vi "Camera_QR Code Detection.vi"(8 "error in (no error)":errorcluster, 10 "QR Code Detection":T1, 11 "SRV In":refnum<k5>) -> (0 "error out":errorcluster, 3 "SRV Out":refnum<k5>)   [LabVIEW 2014]
doc: "Enables/disables the QR Code detection.\n\n\nAuthor: Mike Schultz"
uses:
  ImageProcessing/QR Code Detection Radio Buttons.ctl
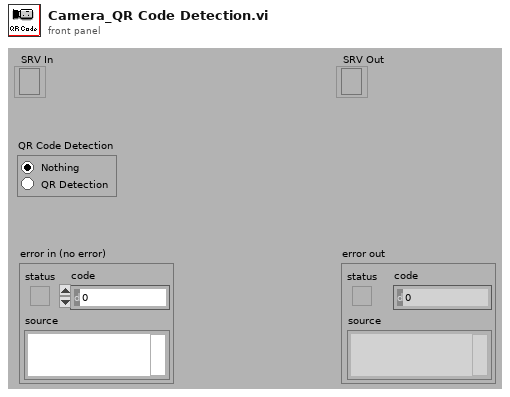
[diagram p1: front panel]
types:
  T1 = typedef "QR Code Detection Radio Buttons.ctl" = enum32{"Nothing", "QR Detection"}
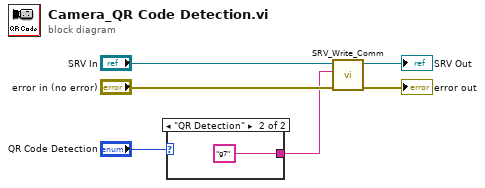
[diagram p0: block diagram]
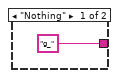
[diagram p2: hidden frame]
diagram:
  n1 = case shown="\"QR Detection\"" "QR Code Detection" {
    tunnel: ["g_" ("Command Sent") "g7" ("Command Sent")] -> w1
    frame "Nothing" {
    }
    frame "QR Detection" {
    }
  }
  n2 = call "SRV_Write_Comm.vi"("error in (no error)"="error in (no error)", "Command Sent"=w1, "SRV In"="SRV In") -> ("error out"=→"error out":errorcluster, "SRV Out"=→"SRV Out":refnum<k5>)  [unwired: 6 in, 1 out]
